vi "Config.Global.vi"() -> ()   [LabVIEW 2016]
uses:
  EventLog/EventLog.Gui.Sets.ctl
  EventLog/EventLog.EventLevelOperatorGui.ctl
  Sequence/Sequence.UserData.ctl
  Sequence/Sequence.MainMode.ctl
  Gui/MainGui.TestOptions.ctl
panel:
  in  "ProdArmMode":bool
  in  "IgnoreWabcoNoFormat":bool
  in  "ArchiverDaysTdms":dbl=365.0
  in  "ArchiverDaysImages":dbl=90.0
  in  "TotalCounter2":u32
  in  "Station2":string
  in  "Station1":string
  in  "Password.DMCConfig":string="81dc9bdb52d04dc20036dbd8313ed055"
  in  "ThresholdLimitB":u8=10
  in  "IgnoreTuning":bool
  in  "ThresholdLimitA":u8=10
  in  "Archiver":bool
  in  "TotalCounter1":u32
  in  "Password":string="81dc9bdb52d04dc20036dbd8313ed055"
  in  "UserSets":T1
  in  "LogsOptions":T4={"IncludeBegin"=FALSE, "dtm_Begin"=timestamp(0 s since 1904-01-01), "IncludeEnd"=FALSE, "dtm_End"=timestamp(0 s since 1904-01-01), "Events Level Operator"=enum.">=", "Level"=1, "Source"=1, "SearchText"="", "Freeze"=FALSE} caption="Event.Sets" {"Source" items=["Scanner Prod"]; "Level" items=["Warning"]; "dtm_End" format="%<%.1X\n%x>T"; "dtm_Begin" format="%<%.1X\n%x>T"}
  in  "Language":string
  in  "Simulator":bool
  in  "Touchpanel":bool
  in  "Transparency":u8=10
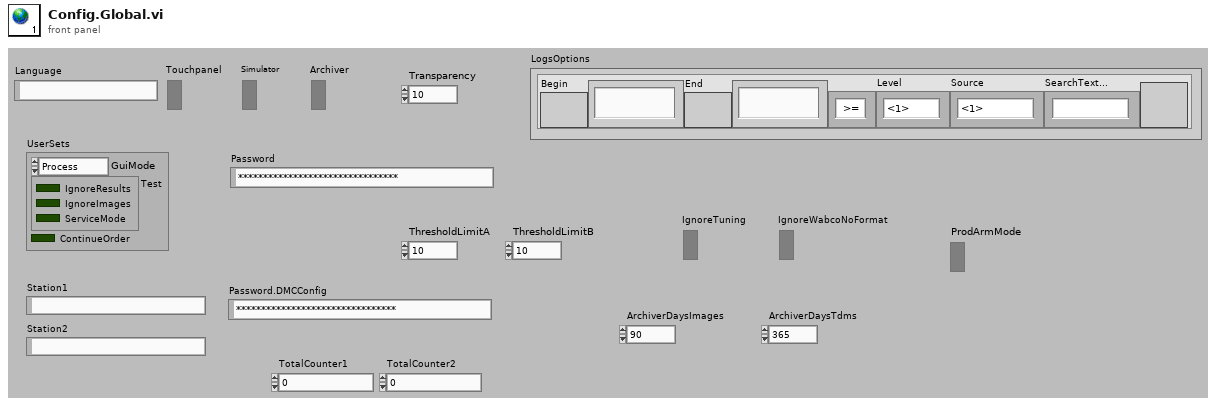
[diagram p1: front panel]
types:
  T1 = typedef "Sequence.UserData.ctl" = cluster{"GuiMode":T2, "Test":T3, "ContinueOrder":bool}
  T2 = typedef "Sequence.MainMode.ctl" = enum16{"Process", "Base", "Order", "Manual", "Logs", "Results", "Stats", "DMC Config"}
  T3 = typedef "MainGui.TestOptions.ctl" = cluster{"IgnoreResults":bool, "IgnoreImages":bool, "ServiceMode":bool}
  T4 = typedef "EventLog.Gui.Sets.ctl" = cluster{"IncludeBegin":bool, "dtm_Begin":timestamp, "IncludeEnd":bool, "dtm_End":timestamp, "Events Level Operator":T5, "Level":u16, "Source":u16, "SearchText":string, "Freeze":bool}
  T5 = typedef "EventLog.EventLevelOperatorGui.ctl" = enum16{">=", "=", "<="}
diagram:
